vi "Inspect VI.vi"(8 "error in (no error)":errorcluster, 11 "VI Path":path=path "C:/dev/SoL/sol-word-search/Scorer (2024Q1)/Scorer/Naughty VI Test.vi") -> (0 "error out":errorcluster, 2 "Issues":string[](array[string]))   [LabVIEW 2024, in "Word Search Scorer.lvlib"]
uses:
  Word Search Scorer.lvlib
  <vilib>/Utility/traverseref.llb/TRef TravTarget.ctl
  <vilib>/Utility/traverseref.llb/VI Scripting - Traverse.lvlib
panel:
  out "Style":string
  out "SubVIs":path[](array[path])
  out "Functions":string[](array[string])
  out "Unhandled Classes":string[](array[string])
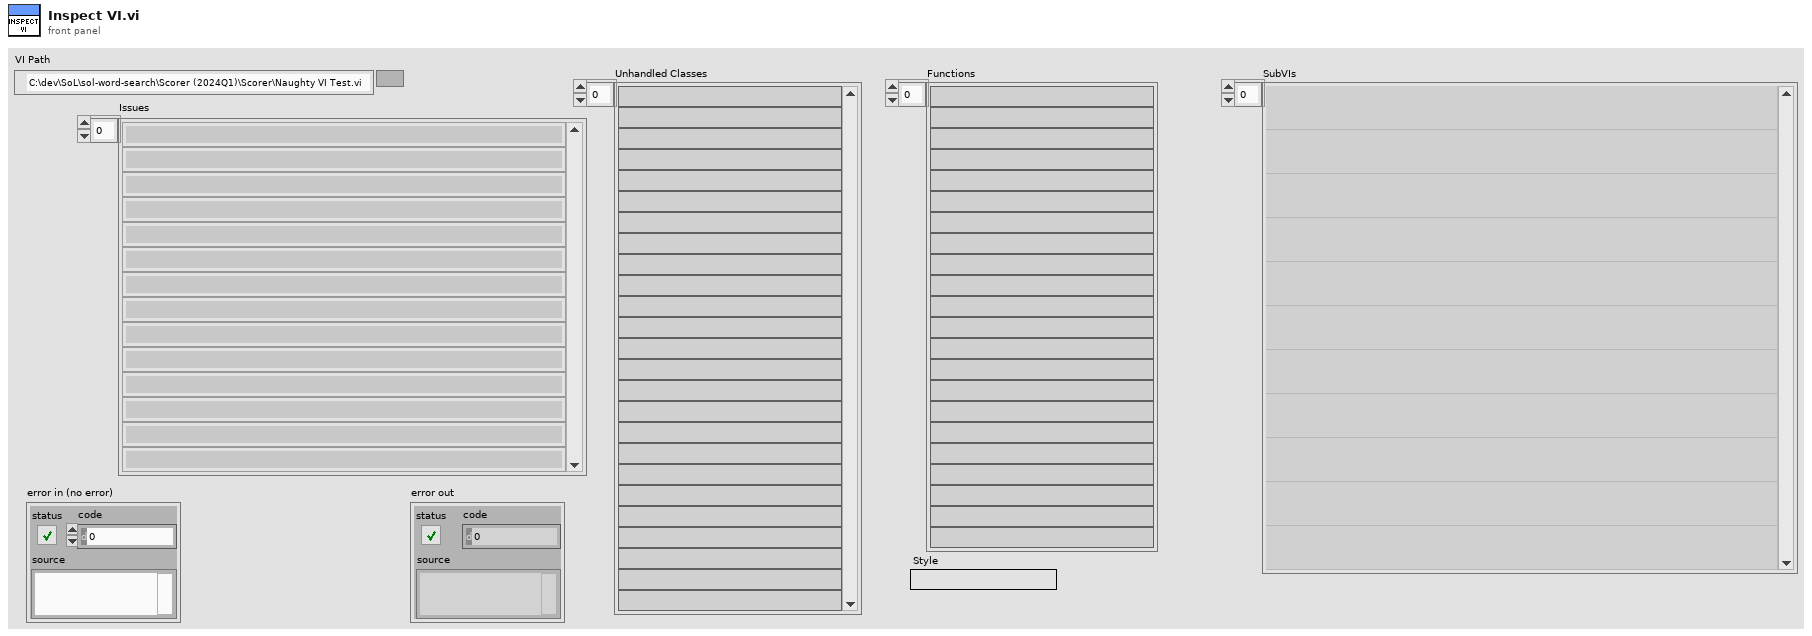
[diagram p1: front panel]
types:
  T1 = typedef "TRef TravTarget.ctl" = enum16{"FP", "BD", "Other"}
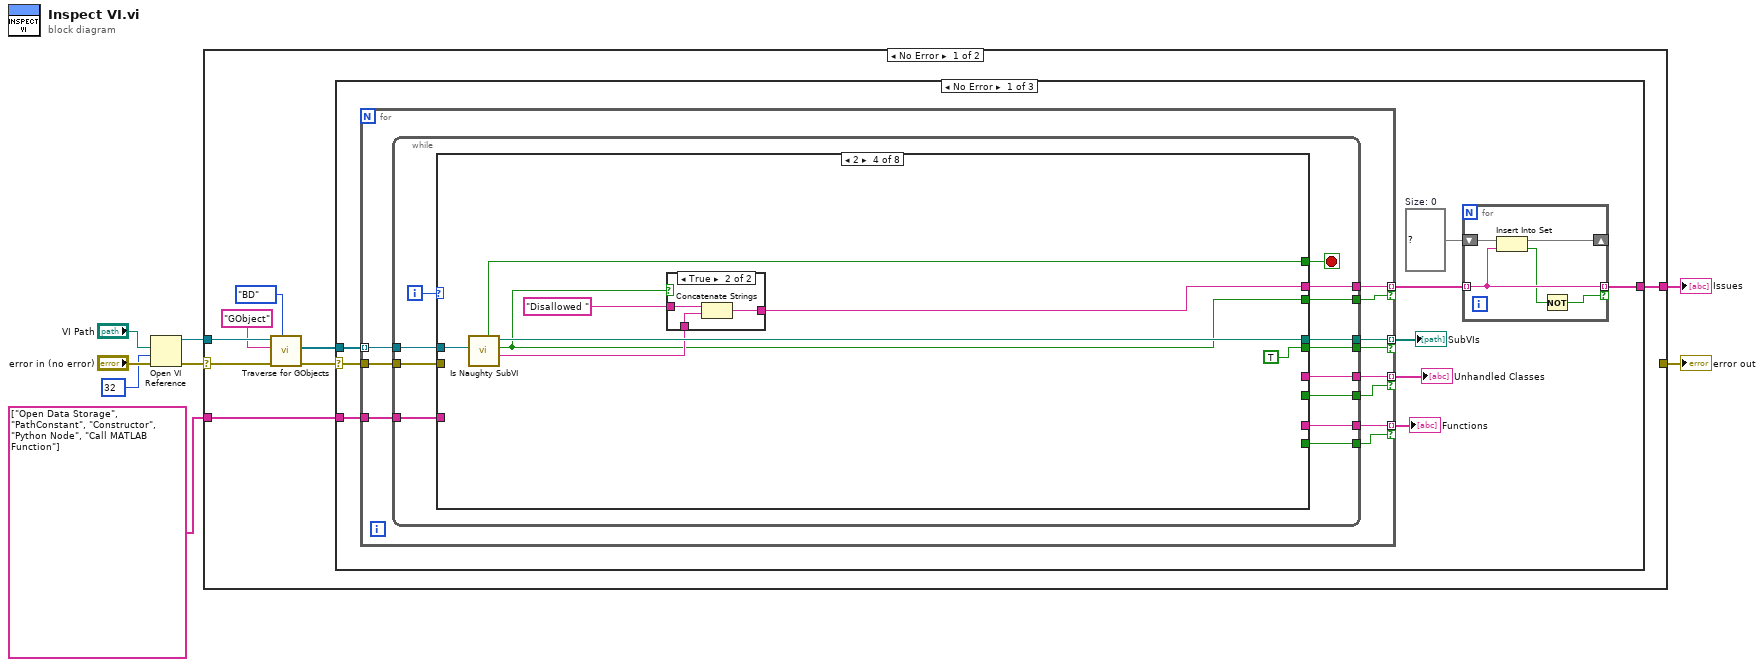
[diagram p0: block diagram]
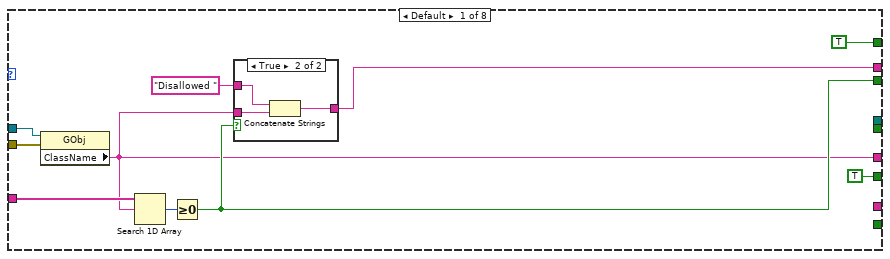
[diagram p2: hidden frame]
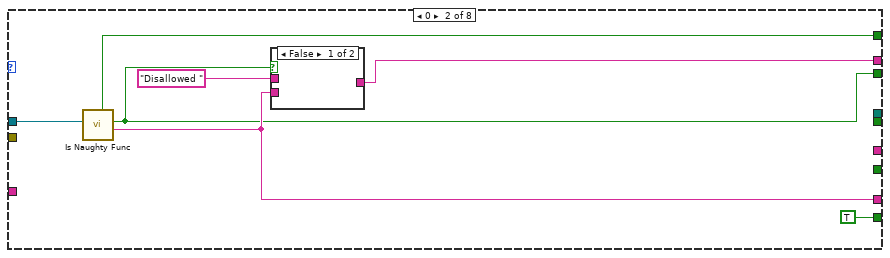
[diagram p4: hidden frame]
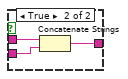
[diagram p5: hidden frame]
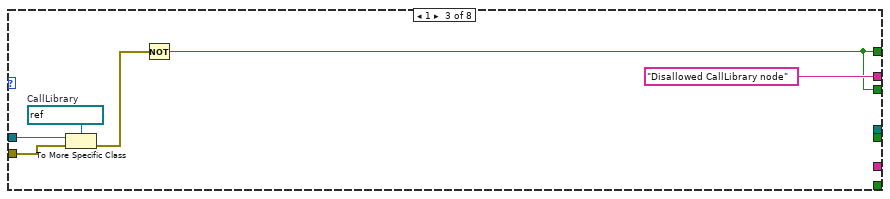
[diagram p6: hidden frame]
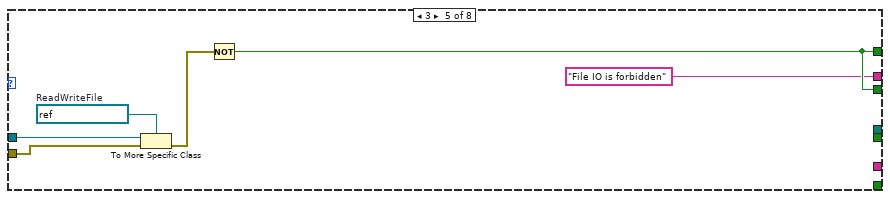
[diagram p8: hidden frame]
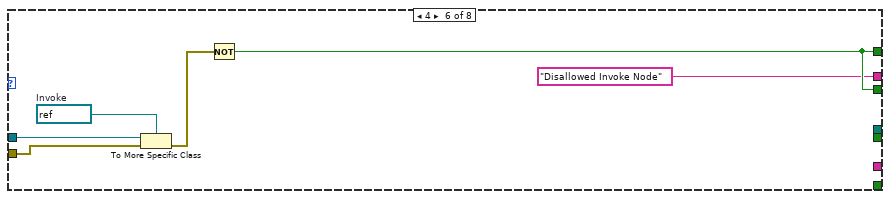
[diagram p9: hidden frame]
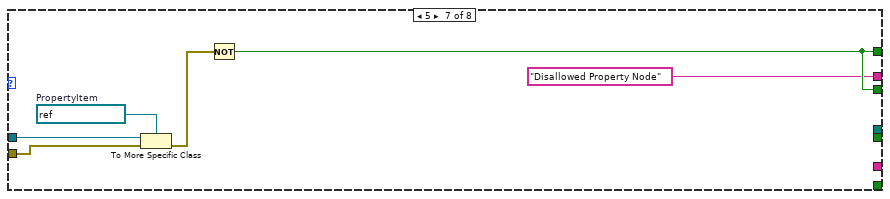
[diagram p10: hidden frame]
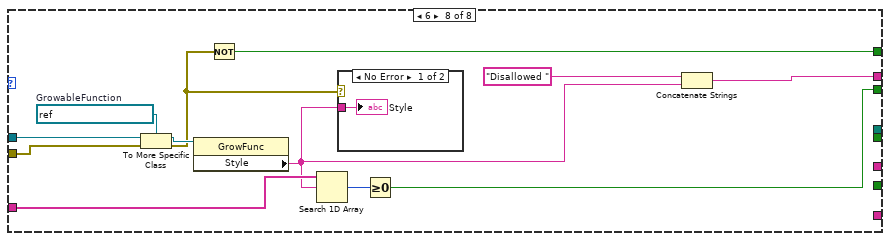
[diagram p11: hidden frame]
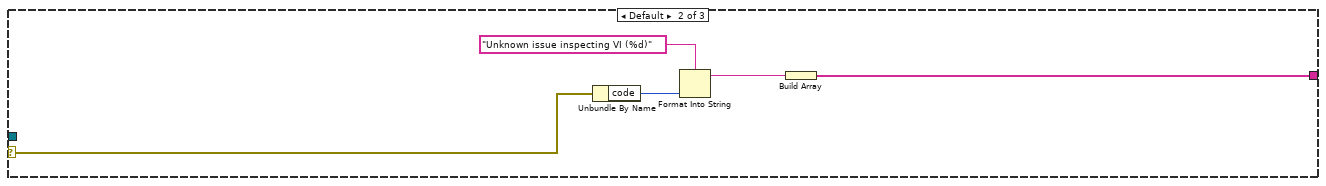
[diagram p13: hidden frame]
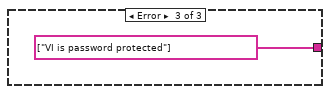
[diagram p14: hidden frame]
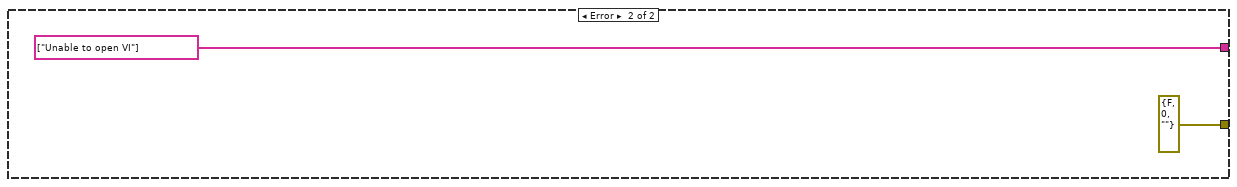
[diagram p15: hidden frame]
diagram:
  n1 = Open VI Reference(vi path="VI Path", options=32, error in (no error)="error in (no error)") -> (vi reference=w4:refnum<vi>, error out=w5:errorcluster)  [unwired: 3 in]
  n2 = case shown="No Error" w5 {
    selector: w5 -> [w15 _]
    tunnel: w4 -> [w16 _]
    tunnel: [w10 string[] ["Unable to open VI"]] -> w3
    tunnel: [_ errorcluster {"status"=FALSE, "code"=0, "source"=""} ("error constant")] -> w2
    tunnel: string[] ["Open Data Storage", "PathConstant", "Constructor", "Python Node", "Call MATLAB Function"] -> [w9 _]
    frame No Error {
      n3 = call <vilib>:"Traverse for GObjects.vi"("Traverse Target"=TRef_TravTarget."BD", "error in (no error)"=w15, "Class Name"="GObject", "VI Refnum"=w16) -> ("error out"=w11:errorcluster, "References"=w12:refnum<vi>[])  [unwired: 4 in, 2 out]
      n4 = case shown="No Error" w11 {
        selector: w11 -> [w24 w126 _]
        tunnel: w12 -> [w25 _ _]
        tunnel: [w17 w127 string[] ["VI is password protected"]] -> w10
        tunnel: w9 -> [w20 _ _]
        frame No Error {
          w18 = set{string} {}  # Size: 0
          n5 = for {
            tunnel: w25 -> [w41] mode=indexing
            tunnel: w24 -> [w40]
            tunnel: [w39] -> w23 mode=indexing if=w38
            tunnel: [w37] -> w22 mode=indexing if=w36
            tunnel: [w35] -> w19 mode=indexing if=w34
            tunnel: [w33] -> w21 mode=indexing if=w32
            tunnel: w20 -> [w31]
            n6 = while {
              tunnel: w41 -> [w52]
              tunnel: w40 -> [w51]
              tunnel: [w50] -> w39
              tunnel: [w49] -> w38
              tunnel: [w48] -> w37
              tunnel: [w47] -> w36
              tunnel: [w46] -> w35
              tunnel: [w45] -> w34
              tunnel: [w44] -> w33
              tunnel: [w43] -> w32
              tunnel: w31 -> [w42]
              i -> [w54]
              stop <- w53 stop-if-true
              n7 = case shown="2" w54 {
                tunnel: [TRUE w68 w78 w89 w96 w102 w108 w117] -> w53
                tunnel: w52 -> [w62 w73 w83 w84 w100 w106 w112 w124]
                tunnel: w51 -> [w63 _ w82 _ w99 w105 w111 w123]
                tunnel: [w56 _ _ _ _ _ _ _] -> w50
                tunnel: [TRUE _ _ _ _ _ _ _] -> w49
                tunnel: [_ w71 _ _ _ _ _ _] -> w48
                tunnel: [_ TRUE _ _ _ _ _ _] -> w47
                tunnel: [w55 w70 "Disallowed CallLibrary node" w86 "File IO is forbidden" "Disallowed Invoke Node" "Disallowed Property Node" w114] -> w46
                tunnel: [w58 w69 w78 w85 w96 w102 w108 w116] -> w45
                tunnel: [_ _ _ w91 _ _ _ _] -> w44
                tunnel: [_ _ _ TRUE _ _ _ _] -> w43
                tunnel: w42 -> [w60 _ _ _ _ _ _ w119]
                frame Default {
                  n8 = property class="GObj"(reference=w62, error in=w63) -> ("ClassName"=w56:string)  [unwired: 2 out]
                  n9 = Search 1D Array(1D array=w60, element=w56) -> (index of element=w59:i32)  [unwired: 1 in]
                  n10 = Greater Or Equal To 0?(x=w59) -> (x >= 0?=w58:bool)
                  n11 = case shown="True" w58 {
                    tunnel: "Disallowed " -> [_ w67]
                    tunnel: w56 -> [_ w66]
                    tunnel: [_ w65] -> w55
                    frame False {
                    }
                    frame True {
                      n12 = Concatenate Strings(w67, w66) -> (w65:string)
                    }
                  }
                }
                frame 0 {
                  n13 = call "Is Naughty Func.vi"("GObj Refnum"=w73) -> ("Function"=w71:string, "Naughty Function"=w69:bool, "Is Func"=w68:bool)  [unwired: 8 in]
                  n14 = case shown="False" w69 {
                    tunnel: "Disallowed " -> [_ w77]
                    tunnel: w71 -> [_ w76]
                    tunnel: [_ w75] -> w70
                    frame False {
                    }
                    frame True {
                      n15 = Concatenate Strings(w77, w76) -> (w75:string)
                    }
                  }
                }
                frame 1 {
                  w81 = refnum<vi> refnum  # CallLibrary
                  n16 = To More Specific Class(target class=w81, reference=w83, error in=w82) -> (error out=w80:errorcluster)  [unwired: 1 out]
                  n17 = Not(x=w80) -> (.not. x?=w78:bool)
                }
                frame 2 {
                  n18 = call "Is Naughty SubVI.vi"("GObj Refnum"=w84) -> ("SubVI"=w87:string, "Naughty SubVI"=w85:bool, "VIPath"=w91:path, "Is SubVI"=w89:bool)  [unwired: 7 in]
                  n19 = case shown="True" w85 {
                    tunnel: "Disallowed " -> [_ w94]
                    tunnel: w87 -> [_ w93]
                    tunnel: [_ w92] -> w86
                    frame False {
                    }
                    frame True {
                      n20 = Concatenate Strings(w94, w93) -> (w92:string)
                    }
                  }
                }
                frame 3 {
                  w98 = refnum<vi> refnum  # ReadWriteFile
                  n21 = To More Specific Class(target class=w98, reference=w100, error in=w99) -> (error out=w97:errorcluster)  [unwired: 1 out]
                  n22 = Not(x=w97) -> (.not. x?=w96:bool)
                }
                frame 4 {
                  w104 = refnum<vi> refnum  # Invoke
                  n23 = To More Specific Class(target class=w104, reference=w106, error in=w105) -> (error out=w103:errorcluster)  [unwired: 1 out]
                  n24 = Not(x=w103) -> (.not. x?=w102:bool)
                }
                frame 5 {
                  w110 = refnum<vi> refnum  # PropertyItem
                  n25 = To More Specific Class(target class=w110, reference=w112, error in=w111) -> (error out=w109:errorcluster)  [unwired: 1 out]
                  n26 = Not(x=w109) -> (.not. x?=w108:bool)
                }
                frame 6 {
                  w122 = refnum<vi> refnum  # GrowableFunction
                  n27 = To More Specific Class(target class=w122, reference=w124, error in=w123) -> (specific class reference=w120:refnum<vi>, error out=w115:errorcluster)
                  n28 = property class="GrowFunc"(reference=w120) -> ("Style"=w113:string)  [unwired: 1 in, 2 out]
                  n29 = Not(x=w115) -> (.not. x?=w117:bool)
                  n30 = Search 1D Array(1D array=w119, element=w113) -> (index of element=w118:i32)  [unwired: 1 in]
                  n31 = case shown="No Error" w115 {
                    tunnel: w113 -> [w125 _]
                    frame No Error {
                      "Style" <- w125
                    }
                    frame Error {
                    }
                  }
                  n32 = Greater Or Equal To 0?(x=w118) -> (x >= 0?=w116:bool)
                  n33 = Concatenate Strings("Disallowed ", w113) -> (w114:string)
                }
              }
            }
          }
          "Unhandled Classes" <- w23
          "Functions" <- w22
          "SubVIs" <- w21
          n34 = for {
            tunnel: w19 -> [w28] mode=indexing
            shift-right: [w29] -> _
            shift-left: w18 -> [w30]
            tunnel: [w28] -> w17 mode=indexing if=w26
            n35 = Insert Into Set(10:w28, 11:w30) -> (2:w27:bool, 3:w29:set{string})
            n36 = Not(x=w27) -> (.not. x?=w26:bool)
          }
        }
        frame Default {
          n37 = Unbundle By Name(w126) -> ("code"=w129:i32)
          n38 = Format Into String(format string="Unknown issue inspecting VI (%d)", w129) -> (resulting string=w128:string)  [unwired: 2 in, 1 out]
          n39 = Build Array(w128) -> (w127:string[])
        }
        frame Error {
        }
      }
    }
    frame Error {
    }
  }
  "error out" <- w2
  "Issues" <- w3
